vi "main.vi"() -> ()   [LabVIEW 2017]
doc: "This template is for the Queued Message Handler design pattern.\n\nThe Event Handling Loop generates messages based on user interface actions.\n\nThe Message Handling Loop processes messages generated by the Event Handling Loop, or by other messages. The messages are string values, so new messages can be added easily to the Message Cases case structure in the Message Handling Loop. Each message cluster can also provide an optional value for Message Data, which is a variant that can be converted to whatever message-specific data is required."
uses:
  controls/UI Data.ctl
  support/Message Queue/Message Queue.lvlib
  <vilib>/Utility/error.llb/Error Cluster From Error Code.vi
  support/User Event - Stop/User Event - Stop.lvlib
  support/Message Queue/Enqueue Message (Single).vi
  <vilib>/ErrorRing/Error Ring.xnode
  logger/logger.lvlib
  worker/worker.lvlib
panel:
  out "Status":string
  in  "Exit":bool
  # "Worker"
  # "Hardware"
  # "Task"
  # "Read Analog"
  # "NiHardware / Sim"
  # "Read Analog Task"
  # "Write Analog"
  # "NiHardware / Sim"
  # "Write Analog Task"
  # "Read Digital"
  # "NiHardware / Sim"
  # "Read Digital Task"
  # "Write Digital"
  # "NiHardware / Sim"
  # "Write Digital Task"
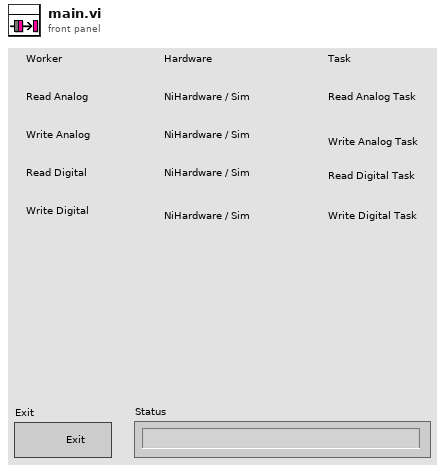
[diagram p1: front panel]
types:
  T1 = typedef "UI Data.ctl" = cluster{"Boolean":bool, "String":string, "Numeric":dbl, "Data Display Ref":refnum<vi>, "Exit Button Ref":refnum<vi>}
  T2 = typedef "Notifiers.ctl" = cluster{"TCPServerExit":refnum<notifier>, "RequestProcesscorExit":refnum<notifier>, "AnalogReadWorkerrExit":refnum<notifier>, "AnalogWriteWorkerrExit":refnum<notifier>, "DigitalReadWorkerrExit":refnum<notifier>, "DigitalWriteWorkerrExit":refnum<notifier>}
  T3 = typedef "Message Queue.lvlib/All Message Queues.ctl" = cluster{"MHL":refnum<queue>, "TCPServerLoop":refnum<queue>, "RequestProcessorLoop":refnum<queue>, "AnalogReadWorkerLoop":refnum<queue>, "AnalogWriteWorkerLoop":refnum<queue>, "DigitalReadWorkerLoop":refnum<queue>, "DigitalWriteWorkerLoop":refnum<queue>}
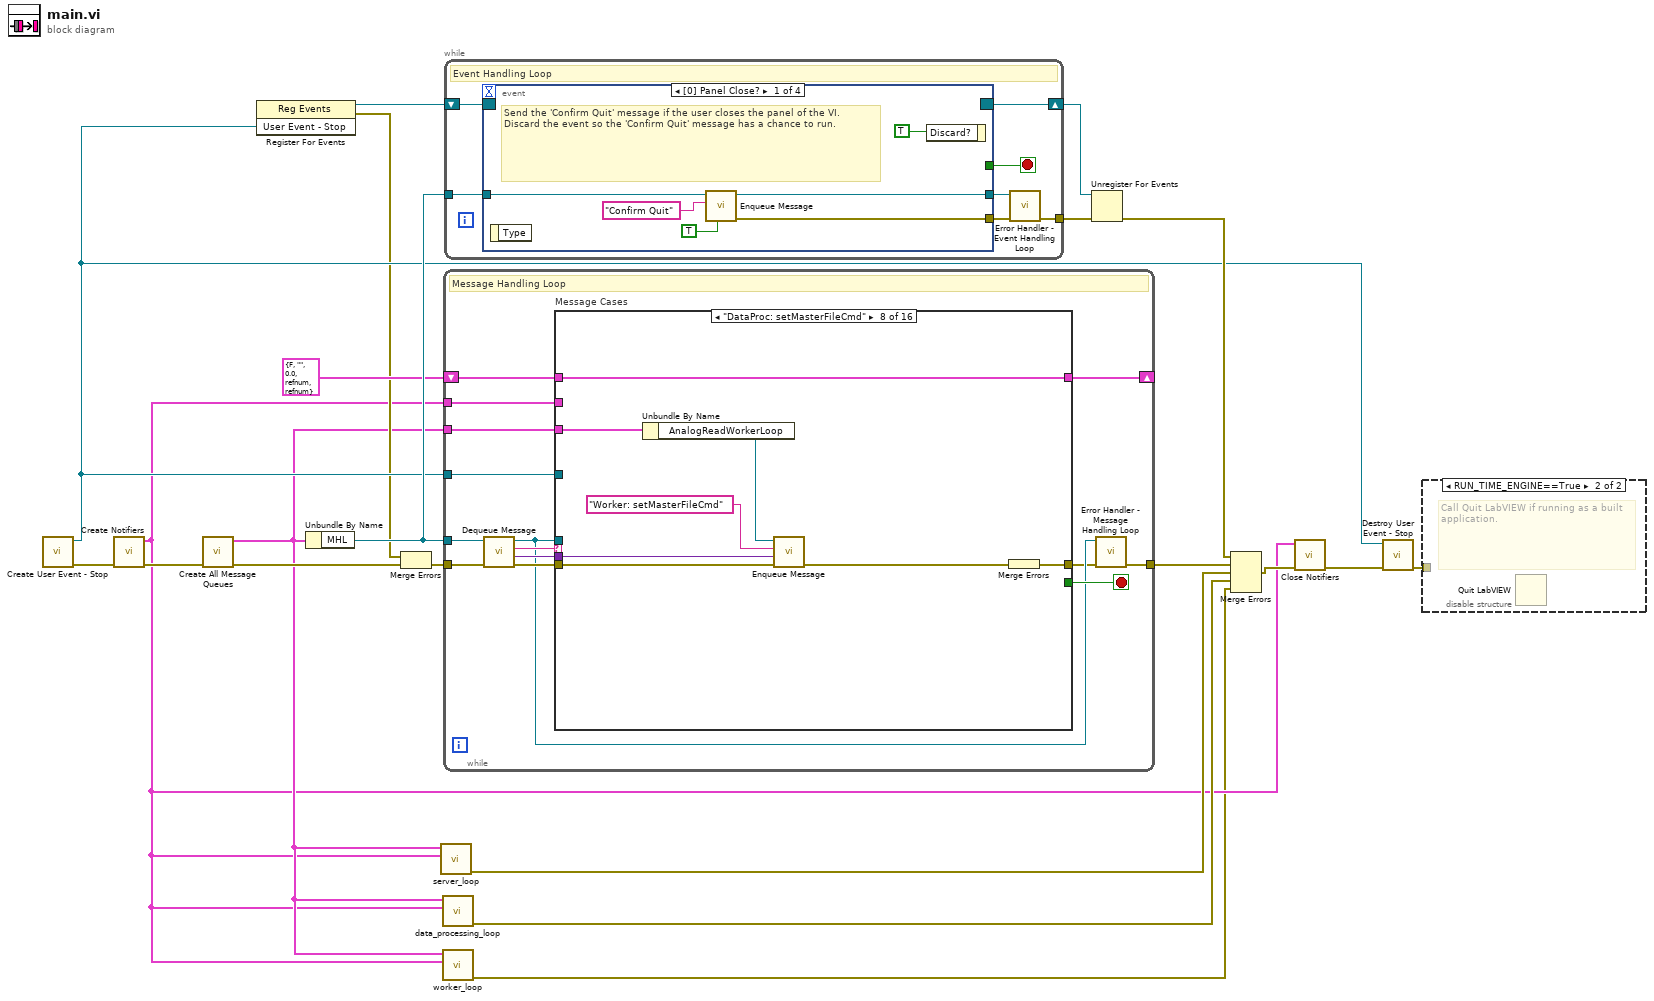
[diagram p0: block diagram]
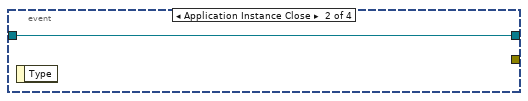
[diagram p3: hidden frame]
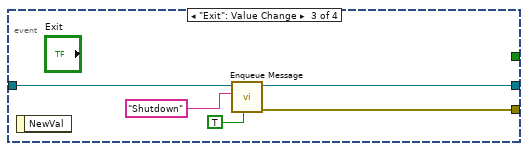
[diagram p4: hidden frame]
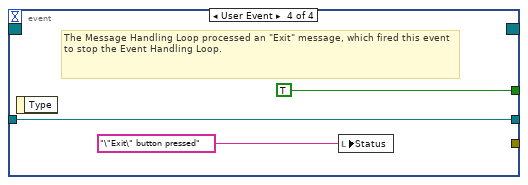
[diagram p5: hidden frame]
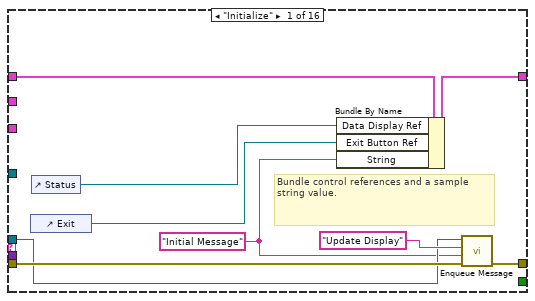
[diagram p6: hidden frame]
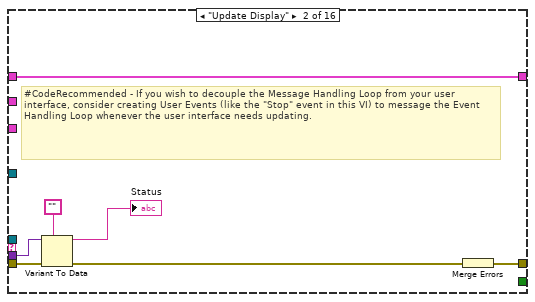
[diagram p7: hidden frame]
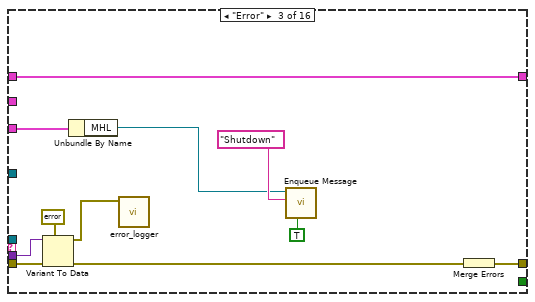
[diagram p8: hidden frame]
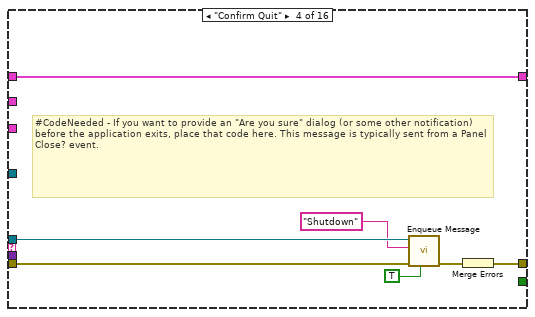
[diagram p9: hidden frame]
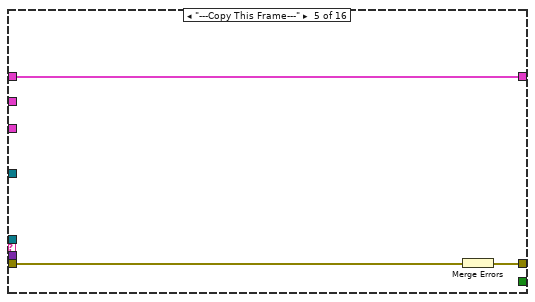
[diagram p10: hidden frame]
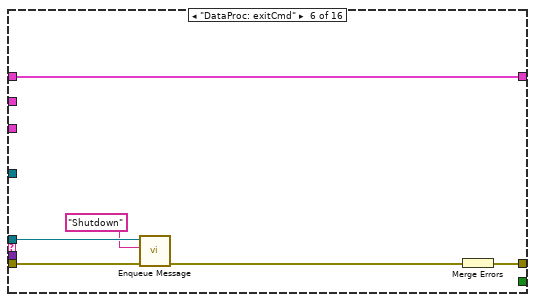
[diagram p11: hidden frame]
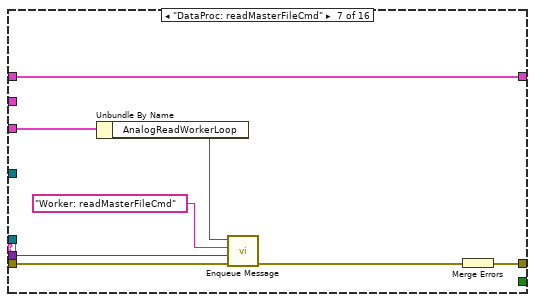
[diagram p12: hidden frame]
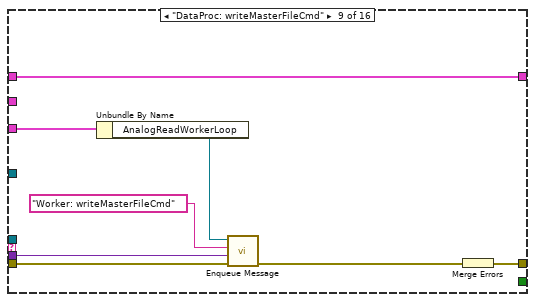
[diagram p13: hidden frame]
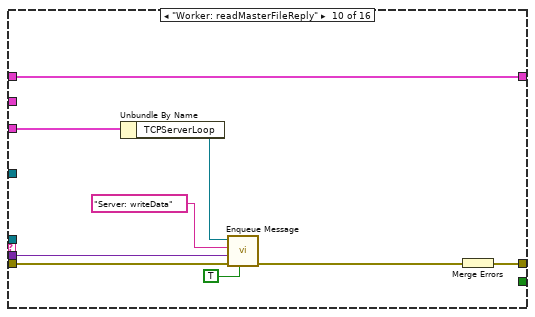
[diagram p14: hidden frame]
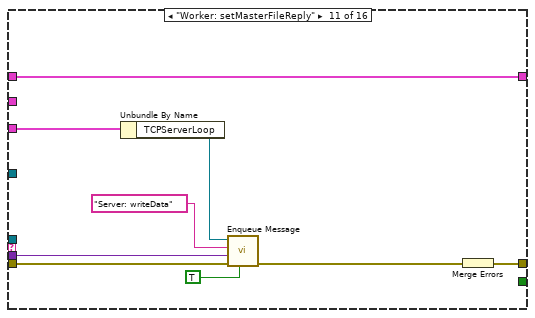
[diagram p15: hidden frame]
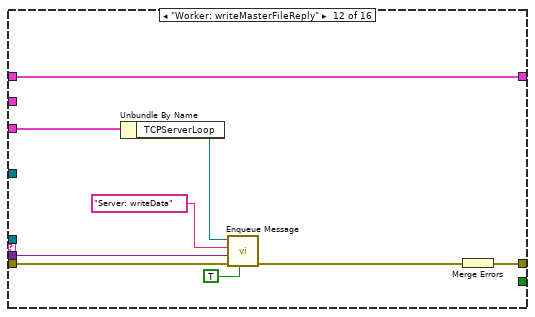
[diagram p16: hidden frame]
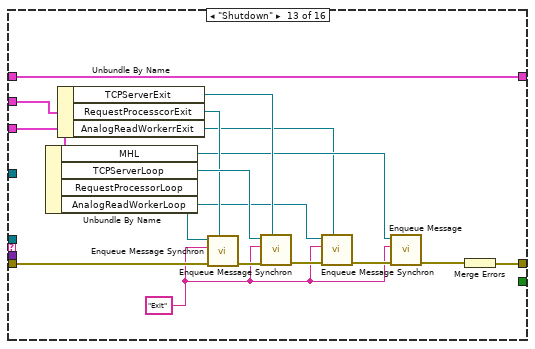
[diagram p17: hidden frame]
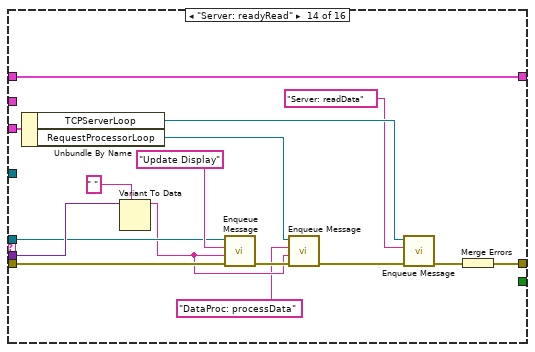
[diagram p18: hidden frame]
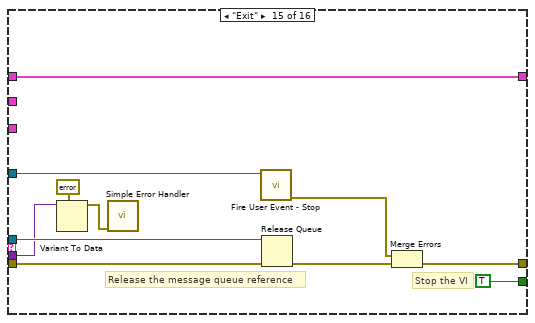
[diagram p19: hidden frame]
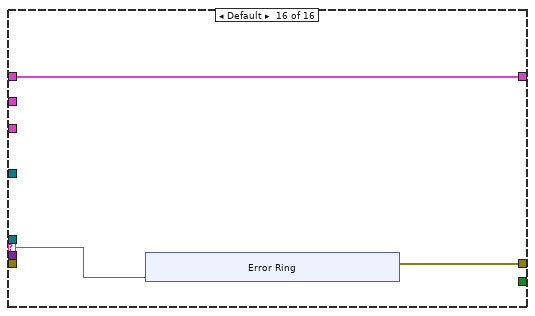
[diagram p20: hidden frame]
diagram:
  n1 = call "Create User Event - Stop.vi"() -> ("error out"=w8:errorcluster, "User Event - Stop"=w12:refnum<user-event>)  [unwired: 10 in]
  n2 = call "Create Notifiers.vi"("error in"=w8) -> ("error out"=w7:errorcluster, "Notifiers"=w2:T2)  [unwired: 9 in]
  n3 = call "Create All Message Queues.vi"("error in (no error)"=w7) -> ("error out"=w21:errorcluster, "Message Queues out"=w3:T3)  [unwired: 9 in]
  n4 = register-events(w12) -> (reference out=w13:refnum<event-registration>, error out=w10:errorcluster)  [unwired: 2 in]
  n5 = Unbundle By Name(w3) -> ("MHL"=w19:refnum<queue>)
  n6 = Merge Errors(w10, w21) -> (w11:errorcluster)
  n7 = call "server_loop.vi"("Notifiers"=w2, "Message Queues"=w3) -> ("error out"=w9:errorcluster)  [unwired: 9 in]
  n8 = call "data_processing_loop.vi"("Notifiers"=w2, "Message Queues"=w3) -> ("error out"=w6:errorcluster)  [unwired: 9 in]
  n9 = call "worker_loop.vi"("Notifiers"=w2, "Message Queues"=w3) -> ("error out"=w1:errorcluster)  [unwired: 9 in]
  n10 = while {
    tunnel: w19 -> [w27]
    shift-right: [w34] -> _
    shift-left: T1 {"Boolean"=FALSE, "String"="", "Numeric"=0.0, "Data Display Ref"=refnum, "Exit Button Ref"=refnum} ("Data Cluster") -> [w35]
    tunnel: w12 -> [w32]
    tunnel: w11 -> [w31]
    tunnel: [w25] -> w20
    tunnel: w3 -> [w23]
    tunnel: w2 -> [w22]
    stop <- w33 stop-if-true
    # "Message Handling Loop"
    n11 = call "Dequeue Message.vi"("error in (no error)"=w31, "Message Queue"=w27) -> ("error out"=w30:errorcluster, "Message Data"=w28:variant, "Message"=w29:string, "dup Message Queue"=w26:refnum<queue>)  [unwired: 6 in]
    n12 = case "Message Cases" shown="\"DataProc: setMasterFileCmd\"" w29 {
      selector: w29 -> [_ _ _ _ _ _ _ _ _ _ _ _ _ _ _ w174]
      tunnel: w26 -> [w37 _ _ w65 _ w74 _ _ _ _ _ _ _ w156 w173 _]
      tunnel: w30 -> [w43 w49 w62 w69 w72 w76 w84 w92 w100 w109 w118 w127 w142 w158 w166 _]
      tunnel: [w44 w50 w58 w67 w70 w77 w85 w93 w101 w110 w119 w128 w145 w161 w169 w175] -> w24
      tunnel: w35 -> [w42 w51 w61 w68 w71 w78 w86 w94 w102 w111 w120 w129 w146 w162 w172 w176]
      tunnel: [w41 w51 w61 w68 w71 w78 w86 w94 w102 w111 w120 w129 w146 w162 w172 w176] -> w34
      tunnel: [_ _ _ _ _ _ _ _ _ _ _ _ _ _ TRUE _] -> w33
      tunnel: w28 -> [_ w48 w60 _ _ _ w79 w87 w95 w104 w113 w122 _ w160 w163 _]
      tunnel: w32 -> [_ _ _ _ _ _ _ _ _ _ _ _ _ _ w168 _]
      tunnel: w23 -> [_ _ w53 _ _ _ w82 w90 w98 w107 w116 w125 w144 w155 _ _]
      tunnel: w22 -> [_ _ _ _ _ _ _ _ _ _ _ _ w143 _ _ _]
      frame "Initialize" {
        w36 = "Initial Message" ("Initial Message")
        # "Bundle control references and a sample string value."
        # "Initialize - All initialization work should take place in this message, since other loops can potentially enqueue messages that execute immediately after this one."
        n13 = control-ref of="Exit"() -> (w39:refnum<vi>)
        n14 = control-ref of="Status"() -> (w40:refnum<vi>)
        n15 = Bundle By Name(cluster=w42, "Data Display Ref"=w40, "Exit Button Ref"=w39, "String"=w36) -> (w41:T1)
        n16 = call-poly "Enqueue Message.vi"("error in (no error)"=w43, "Message Data"=w36, "Message"="Update Display", "Message Queue"=w37) -> ("error out"=w44:errorcluster)  [unwired: 6 in, 1 out]
      }
      frame "Update Display" {
        # "#CodeRecommended - If you wish to decouple the Message Handling Loop from your user interface, consider creating User Events (like the \"Stop\" event in this VI) to message the Event Handling Loop whenever the user interface needs updating."
        # "Update Display - Convert the message data to a string to display in the Data Display indicator."
        n17 = Variant To Data(error in=w49, type="", Variant=w48) -> (data=→"Status":string, error out=w46:errorcluster)
        n18 = Merge Errors(w46) -> (w50:errorcluster)
      }
      frame "Error" {
        # "Error - Display an error dialog. This message is sent by the \"Error Handler\" VIs at the end of other loops in this application."
        n19 = Variant To Data(error in=w62, type=errorcluster {"status"=FALSE, "code"=0, "source"=""} ("error constant"), Variant=w60) -> (data=w57:errorcluster, error out=w56:errorcluster)
        n20 = Unbundle By Name(w53) -> ("MHL"=w52:refnum<queue>)
        n21 = call "error_logger.vi"("error in (no error)"=w57) -> ()  [unwired: 11 in]
        n22 = call-poly "Enqueue Message.vi"("Priority Message? (F)"=TRUE, "Message"="Shutdown", "Message Queue"=w52) -> ()  [unwired: 7 in, 2 out]
        n23 = Merge Errors(w56) -> (w58:errorcluster)
      }
      frame "Confirm Quit" {
        # "#CodeNeeded - If you want to provide an \"Are you sure\" dialog (or some other notification) before the application exits, place that code here. This message is typically sent from a Panel Close? event."
        # "Confirm Quit - Message that can confirm whether or not the user wants to exit the application."
        n24 = call-poly "Enqueue Message.vi"("Priority Message? (F)"=TRUE, "error in (no error)"=w69, "Message"="Shutdown", "Message Queue"=w65) -> ("error out"=w66:errorcluster)  [unwired: 6 in, 1 out]
        n25 = Merge Errors(w66) -> (w67:errorcluster)
      }
      frame "---Copy This Frame---" {
        # "Duplicate this frame when creating new messages.  Change this comment in the duplicated frame to describe this message."
        n26 = Merge Errors(w72) -> (w70:errorcluster)
      }
      frame "DataProc: exitCmd" {
        # "Duplicate this frame when creating new messages.  Change this comment in the duplicated frame to describe this message."
        n27 = call-poly "Enqueue Message.vi"("error in (no error)"=w76, "Message"="Shutdown", "Message Queue"=w74) -> ("error out"=w75:errorcluster)  [unwired: 7 in, 1 out]
        n28 = Merge Errors(w75) -> (w77:errorcluster)
      }
      frame "DataProc: readMasterFileCmd" {
        # "Duplicate this frame when creating new messages.  Change this comment in the duplicated frame to describe this message."
        n29 = Unbundle By Name(w82) -> ("AnalogReadWorkerLoop"=w81:refnum<queue>)
        n30 = call-poly "Enqueue Message.vi"("error in (no error)"=w84, "Message Data"=w79, "Message"="Worker: readMasterFileCmd", "Message Queue"=w81) -> ("error out"=w83:errorcluster)  [unwired: 6 in, 1 out]
        n31 = Merge Errors(w83) -> (w85:errorcluster)
      }
      frame "DataProc: setMasterFileCmd" {
        # "Duplicate this frame when creating new messages.  Change this comment in the duplicated frame to describe this message."
        n32 = Unbundle By Name(w90) -> ("AnalogReadWorkerLoop"=w89:refnum<queue>)
        n33 = call-poly "Enqueue Message.vi"("error in (no error)"=w92, "Message Data"=w87, "Message"="Worker: setMasterFileCmd", "Message Queue"=w89) -> ("error out"=w91:errorcluster)  [unwired: 6 in, 1 out]
        n34 = Merge Errors(w91) -> (w93:errorcluster)
      }
      frame "DataProc: writeMasterFileCmd" {
        # "Duplicate this frame when creating new messages.  Change this comment in the duplicated frame to describe this message."
        n35 = Unbundle By Name(w98) -> ("AnalogReadWorkerLoop"=w97:refnum<queue>)
        n36 = call-poly "Enqueue Message.vi"("error in (no error)"=w100, "Message Data"=w95, "Message"="Worker: writeMasterFileCmd", "Message Queue"=w97) -> ("error out"=w99:errorcluster)  [unwired: 6 in, 1 out]
        n37 = Merge Errors(w99) -> (w101:errorcluster)
      }
      frame "Worker: readMasterFileReply" {
        # "Duplicate this frame when creating new messages.  Change this comment in the duplicated frame to describe this message."
        n38 = Unbundle By Name(w107) -> ("TCPServerLoop"=w106:refnum<queue>)
        n39 = call-poly "Enqueue Message.vi"("Priority Message? (F)"=TRUE, "error in (no error)"=w109, "Message Data"=w104, "Message"="Server: writeData", "Message Queue"=w106) -> ("error out"=w108:errorcluster)  [unwired: 5 in, 1 out]
        n40 = Merge Errors(w108) -> (w110:errorcluster)
      }
      frame "Worker: setMasterFileReply" {
        # "Duplicate this frame when creating new messages.  Change this comment in the duplicated frame to describe this message."
        n41 = Unbundle By Name(w116) -> ("TCPServerLoop"=w115:refnum<queue>)
        n42 = call-poly "Enqueue Message.vi"("Priority Message? (F)"=TRUE, "error in (no error)"=w118, "Message Data"=w113, "Message"="Server: writeData", "Message Queue"=w115) -> ("error out"=w117:errorcluster)  [unwired: 5 in, 1 out]
        n43 = Merge Errors(w117) -> (w119:errorcluster)
      }
      frame "Worker: writeMasterFileReply" {
        # "Duplicate this frame when creating new messages.  Change this comment in the duplicated frame to describe this message."
        n44 = Unbundle By Name(w125) -> ("TCPServerLoop"=w124:refnum<queue>)
        n45 = call-poly "Enqueue Message.vi"("Priority Message? (F)"=TRUE, "error in (no error)"=w127, "Message Data"=w122, "Message"="Server: writeData", "Message Queue"=w124) -> ("error out"=w126:errorcluster)  [unwired: 5 in, 1 out]
        n46 = Merge Errors(w126) -> (w128:errorcluster)
      }
      frame "Shutdown" {
        w132 = "Exit" ("Message")
        # "Duplicate this frame when creating new messages.  Change this comment in the duplicated frame to describe this message."
        n47 = Unbundle By Name(w144) -> ("MHL"=w136:refnum<queue>, "TCPServerLoop"=w140:refnum<queue>, "RequestProcessorLoop"=w141:refnum<queue>, "AnalogReadWorkerLoop"=w131:refnum<queue>)
        n48 = Unbundle By Name(w143) -> ("TCPServerExit"=w138:refnum<notifier>, "RequestProcesscorExit"=w139:refnum<notifier>, "AnalogReadWorkerrExit"=w130:refnum<notifier>)
        n49 = call "Enqueue Message Synchron.vi"("Notifier"=w139, "error in (no error)"=w142, "Message"=w132, "Message Queue"=w141) -> ("error out"=w137:errorcluster)  [unwired: 6 in, 1 out]
        n50 = call "Enqueue Message Synchron.vi"("Notifier"=w138, "error in (no error)"=w137, "Message"=w132, "Message Queue"=w140) -> ("error out"=w134:errorcluster)  [unwired: 6 in, 1 out]
        n51 = call "Enqueue Message Synchron.vi"("Notifier"=w130, "error in (no error)"=w134, "Message"=w132, "Message Queue"=w131) -> ("error out"=w133:errorcluster)  [unwired: 6 in, 1 out]
        n52 = call-poly "Enqueue Message.vi"("error in (no error)"=w133, "Message"=w132, "Message Queue"=w136) -> ("error out"=w135:errorcluster)  [unwired: 7 in, 1 out]
        n53 = Merge Errors(w135) -> (w145:errorcluster)
      }
      frame "Server: readyRead" {
        # "Duplicate this frame when creating new messages.  Change this comment in the duplicated frame to describe this message."
        n54 = Unbundle By Name(w155) -> ("TCPServerLoop"=w154:refnum<queue>, "RequestProcessorLoop"=w149:refnum<queue>)
        n55 = Variant To Data(type=" ", Variant=w160) -> (data=w148:string)  [unwired: 1 in, 1 out]
        n56 = call-poly "Enqueue Message.vi"("error in (no error)"=w158, "Message Data"=w148, "Message"="Update Display", "Message Queue"=w156) -> ("error out"=w151:errorcluster)  [unwired: 6 in, 1 out]
        n57 = call-poly "Enqueue Message.vi"("error in (no error)"=w151, "Message Data"=w148, "Message"="DataProc: processData", "Message Queue"=w149) -> ("error out"=w150:errorcluster)  [unwired: 6 in, 1 out]
        n58 = call-poly "Enqueue Message.vi"("error in (no error)"=w150, "Message"="Server: readData", "Message Queue"=w154) -> ("error out"=w152:errorcluster)  [unwired: 7 in, 1 out]
        n59 = Merge Errors(w152) -> (w161:errorcluster)
      }
      frame "Exit" {
        # "Stop the VI"
        # "Release the message queue reference"
        # "Exit - Exit the application."
        n60 = Variant To Data(type=errorcluster {"status"=FALSE, "code"=0, "source"=""} ("error constant"), Variant=w163) -> (data=w164:errorcluster)  [unwired: 1 in, 1 out]
        n61 = call <vilib>:"Simple Error Handler.vi"("error in (no error)"=w164) -> ()  [unwired: 4 in, 5 out]
        n62 = call "Fire User Event - Stop.vi"("User Event - Stop"=w168) -> ("error out"=w167:errorcluster)  [unwired: 10 in]
        n63 = Release Queue(queue=w173, error in (no error)=w166) -> (error out=w170:errorcluster)  [unwired: 1 in, 2 out]
        n64 = Merge Errors(w167, w170) -> (w169:errorcluster)
      }
      frame Default {
        # "'Default' case only runs if there is a message that isn't defined in any of the other cases.  Output a programming error."
        n65 = xnode "Error Ring"("parameter 0"=w174) -> ("error out"=w175:errorcluster)
      }
    }
    n66 = call "Error Handler - Message Handling Loop.vi"("error in (no error)"=w24, "Message Queue"=w26) -> ("dup error in"=w25:errorcluster)  [unwired: 8 in, 1 out]
  }
  n67 = while {
    tunnel: w19 -> [w190]
    shift-right: [w188] -> w17
    shift-left: w13 -> [w189]
    tunnel: [w184] -> w14
    stop <- w186 stop-if-true
    # "Event Handling Loop"
    n68 = event shown="[0] Panel Close?" {
      selector: w189 -> [_ _ _ _]
      dyn-events: [_ _ _ _] -> w188
      timeout: _ -> [_ _ _ _]
      tunnel: [_ _ _ TRUE ("Discard?")] -> w186
      tunnel: w190 -> [w195 w197 w202 w205]
      tunnel: [w194 _ w201 _] -> w187
      tunnel: [w193 w197 w200 w205] -> w185
      event Panel Close? {
        # "Send the 'Confirm Quit' message if the user closes the panel of the VI. Discard the event so the 'Confirm Quit' message has a chance to run."
        n69 = event-data() -> ()  [unwired: 1 in, 1 out]
        n70 = call-poly "Enqueue Message.vi"("Priority Message? (F)"=TRUE, "Message"="Confirm Quit", "Message Queue"=w195) -> ("error out"=w194:errorcluster, "dup Message Queue"=w193:refnum<queue>)  [unwired: 7 in]
        n71 = event-data("Discard?"=TRUE) -> ()  [unwired: 1 in, 1 out]
      }
      event Application Instance Close {
        n72 = event-data() -> ()  [unwired: 1 in, 1 out]
      }
      event "Exit": Value Change {
        n73 = event-data() -> ()  [unwired: 1 in, 1 out]
        n74 = call-poly "Enqueue Message.vi"("Priority Message? (F)"=TRUE, "Message"="Shutdown", "Message Queue"=w202) -> ("error out"=w201:errorcluster, "dup Message Queue"=w200:refnum<queue>)  [unwired: 7 in]
      }
      event User Event {
        # "The Message Handling Loop processed an \"Exit\" message, which fired this event to stop the Event Handling Loop."
        n75 = event-data() -> ()  [unwired: 1 in, 1 out]
        n76 = local write "Status"("\"Exit\" button pressed" ("VI Stopped")) -> ()
      }
    }
    n77 = call "Error Handler - Event Handling Loop.vi"("error in (no error)"=w187, "Message Queue"=w185) -> ("dup error in"=w184:errorcluster)  [unwired: 8 in, 1 out]
  }
  n78 = Unregister For Events(event registration refnum=w17, error in=w14) -> (error out=w18:errorcluster)
  n79 = Merge Errors(w18, w20, w9, w6, w1) -> (w5:errorcluster)
  n80 = call "Close Notifiers.vi"("error in"=w5, "Notifiers"=w2) -> ("error out"=w4:errorcluster)  [unwired: 9 in]
  n81 = call "Destroy User Event - Stop.vi"("error in (no error)"=w4, "User Event - Stop"=w12) -> ("error out"=w15:errorcluster)  [unwired: 9 in]
  n82 = disable-structure shown="RUN_TIME_ENGINE==True" {
    disable-tunnel: w15 -> [_ _]
    frame condition #0 (active) {
    }
    frame condition #1 {
      # "Call Quit LabVIEW if running as a built application."
      n83 = Quit LabVIEW() -> ()  [unwired: 1 in]
    }
  }
